vi "XLP80_EA_Init Devices.vi"(8 "err in":errorcluster, 11 "Simu EAs":T2) -> (0 "Error EAs":T3, 2 "Device Informations":T1)   [LabVIEW 2021]
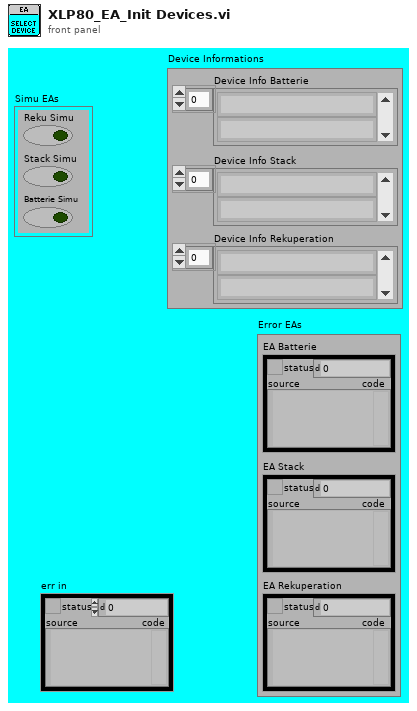
[diagram p1: front panel]
types:
  T1 = cluster{"Device Info Batterie":string[], "Device Info Stack":string[], "Device Info Rekuperation":string[]}
  T2 = cluster{"Reku Simu":bool, "Stack Simu":bool, "Batterie Simu":bool}
  T3 = cluster{"EA Batterie":errorcluster, "EA Stack":errorcluster, "EA Rekuperation":errorcluster}
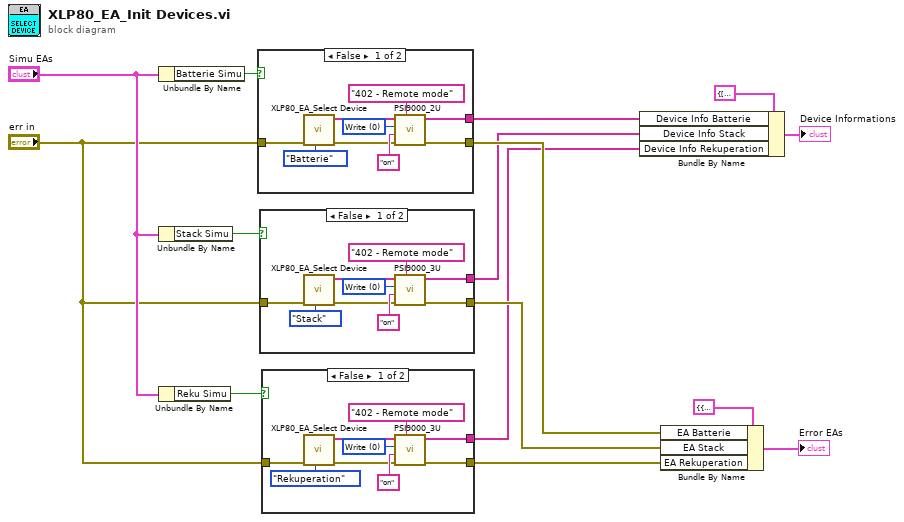
[diagram p0: block diagram]
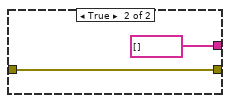
[diagram p2: hidden frame]
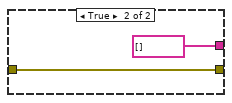
[diagram p3: hidden frame]
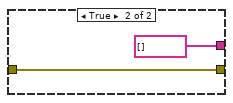
[diagram p4: hidden frame]
diagram:
  n1 = Unbundle By Name("Simu EAs") -> ("Batterie Simu"=w15:bool)
  n2 = Unbundle By Name("Simu EAs") -> ("Stack Simu"=w8:bool)
  n3 = Unbundle By Name("Simu EAs") -> ("Reku Simu"=w5:bool)
  n4 = case shown="False" w15 {
    tunnel: [w21 string[] [] ("Device information out")] -> w9
    tunnel: [w20 w25] -> w13
    tunnel: "err in" -> [w19 w25]
    frame False {
      w23 = u8 0 items=["Write", "Read"] ("Access")
      n5 = call "XLP80_EA_Select Device.vi"("EA Type"=enum16{"Batterie", "Stack", "Rekuperation"}."Batterie", "err in"=w19) -> ("err out"=w18:errorcluster, "Device information"=w17:string[])  [unwired: 8 in]
      n6 = call <instrlib>:"PSI9000_2U.vi"("Command list"="402 - Remote mode", "Error in"=w18, "Value"="on", "Access"=w23, "Device information in"=w17) -> ("Error out"=w20:errorcluster, "Device information out"=w21:string[])  [unwired: 1 in, 2 out]
    }
    frame True {
    }
  }
  n7 = case shown="False" w8 {
    tunnel: [w33 string[] [] ("Device information out")] -> w7
    tunnel: [w32 w36] -> w6
    tunnel: "err in" -> [w31 w36]
    frame False {
      w35 = u8 0 items=["Write", "Read"] ("Access")
      n8 = call "XLP80_EA_Select Device.vi"("EA Type"=enum16{"Batterie", "Stack", "Rekuperation"}."Stack", "err in"=w31) -> ("err out"=w30:errorcluster, "Device information"=w29:string[])  [unwired: 8 in]
      n9 = call <instrlib>:"PSI9000_3U.vi"("Command list"="402 - Remote mode", "Error in"=w30, "Value"="on", "Access"=w35, "Device information in"=w29) -> ("Error out"=w32:errorcluster, "Device information out"=w33:string[])  [unwired: 1 in, 2 out]
    }
    frame True {
    }
  }
  n10 = case shown="False" w5 {
    tunnel: [w44 string[] [] ("Device information out")] -> w1
    tunnel: [w43 w47] -> w2
    tunnel: "err in" -> [w42 w47]
    frame False {
      w46 = u8 0 items=["Write", "Read"] ("Access")
      n11 = call "XLP80_EA_Select Device.vi"("EA Type"=enum16{"Batterie", "Stack", "Rekuperation"}."Rekuperation", "err in"=w42) -> ("err out"=w41:errorcluster, "Device information"=w40:string[])  [unwired: 8 in]
      n12 = call <instrlib>:"PSI9000_3U.vi"("Command list"="402 - Remote mode", "Error in"=w41, "Value"="on", "Access"=w46, "Device information in"=w40) -> ("Error out"=w43:errorcluster, "Device information out"=w44:string[])  [unwired: 1 in, 2 out]
    }
    frame True {
    }
  }
  n13 = Bundle By Name(cluster=T1 {"Device Info Batterie"=[], "Device Info Stack"=[], "Device Info Rekuperation"=[]} ("Device Informations"), "Device Info Batterie"=w9, "Device Info Stack"=w7, "Device Info Rekuperation"=w1) -> (→"Device Informations":T1)
  n14 = Bundle By Name(cluster=T3 {"EA Batterie"={"status"=FALSE, "code"=0, "source"=""}, "EA Stack"={"status"=FALSE, "code"=0, "source"=""}, "EA Rekuperation"={"status"=FALSE, "code"=0, "source"=""}} ("Error EAs"), "EA Batterie"=w13, "EA Stack"=w6, "EA Rekuperation"=w2) -> (→"Error EAs":T3)
